vi "SMS Analysis Interface User Get Data Path.vi"() -> (4 "Transfer Log Path":string, 6 "Image Name":string, 8 "Frames":u32, 10 "Cycles":u16, 15 "Error":errorcluster)   [LabVIEW 2016]
uses:
  Tools/Metadata/Microscope Metadata/Device Metadata Types/Capture Metadata.ctl
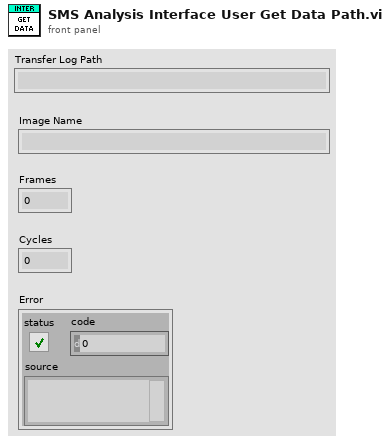
[diagram p1: front panel]
types:
  T1 = typedef "Capture Metadata.ctl" = cluster{"Capture_Exposure_sec":dbl, "Cycles":u16, "Frames":u32, "No_of_Z_Steps":u16, "Z_Step_Size_um":dbl, "Init_Z_Position_um":dbl, "Save_Path":string, "Line_Scan":bool, "Line_Scan_Mode":string}
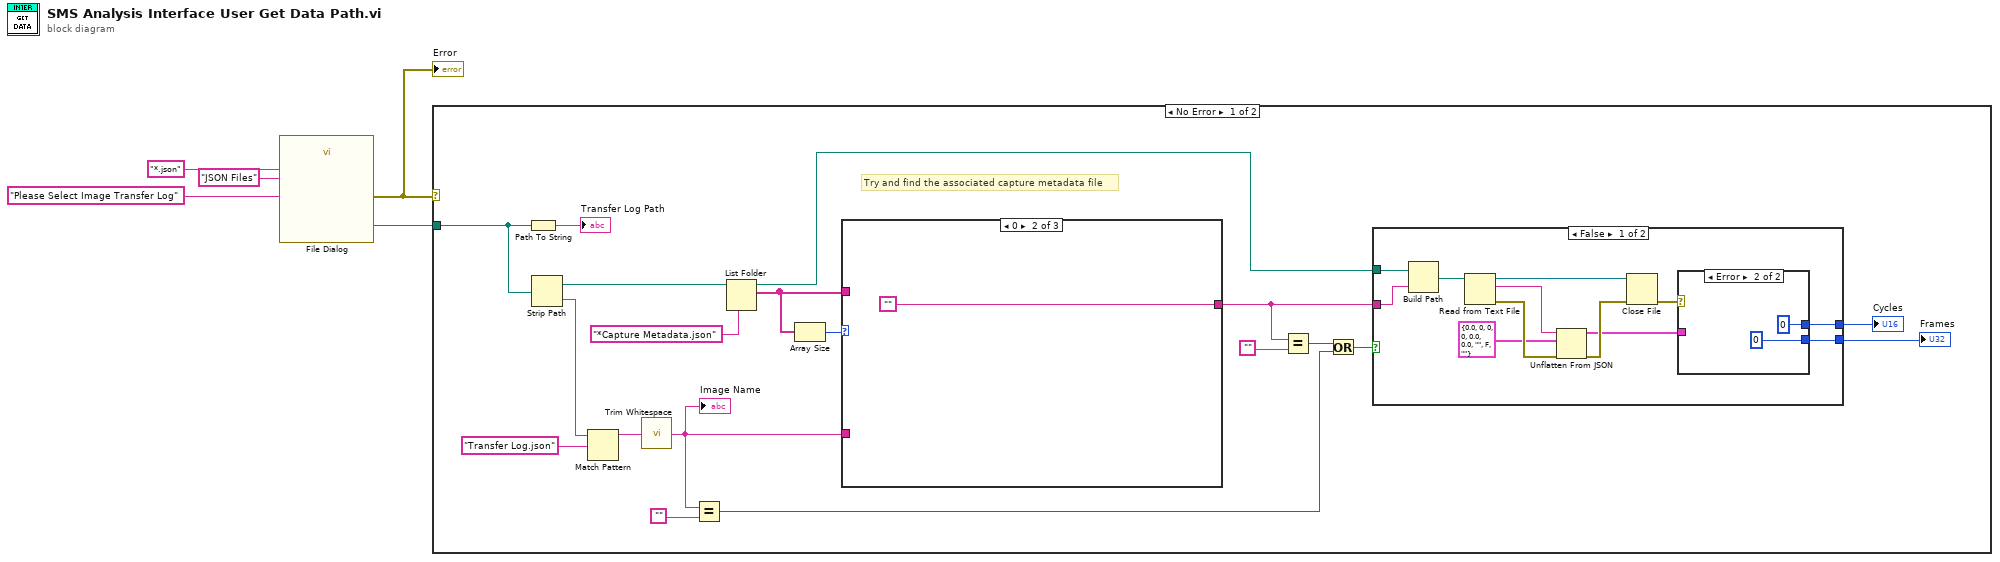
[diagram p0: block diagram]
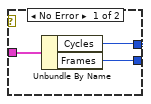
[diagram p2: hidden frame]
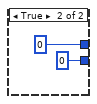
[diagram p3: hidden frame]
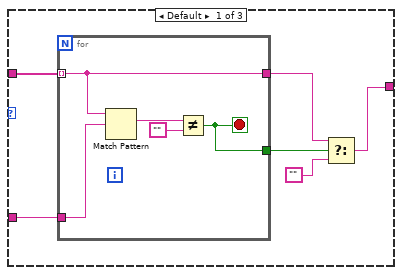
[diagram p4: hidden frame]
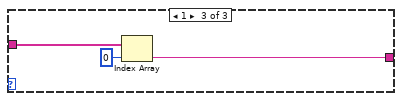
[diagram p5: hidden frame]
diagram:
  n1 = call "File Dialog"("prompt"="Please Select Image Transfer Log", "pattern (all files)"="*.json", "pattern label"="JSON Files") -> ("selected path"=w2:path, "error out"=w1:errorcluster)  [unwired: 9 in, 2 out]
  "Error" <- w1
  n2 = case shown="No Error" w1 {
    tunnel: w2 -> [w23 _]
    frame No Error {
      # "Try and find the associated capture metadata file"
      n3 = Path To String(path=w23) -> (string=→"Transfer Log Path":string)
      n4 = Strip Path(path=w23) -> (stripped path=w22:path, name=w19:string)
      n5 = Match Pattern(string=w19, regular expression="Transfer Log.json") -> (before substring=w18:string)  [unwired: 1 in, 3 out]
      n6 = call <vilib>:"Trim Whitespace.vi"("string"=w18) -> ("trimmed string"=w15:string)  [unwired: 1 in]
      "Image Name" <- w15
      n7 = Equal?(x=w15, y="") -> (x = y?=w11:bool)
      n8 = List Folder(path=w22, pattern="*Capture Metadata.json") -> (path out=w8:path, filenames=w16:string[])  [unwired: 2 in, 2 out]
      n9 = Array Size(array=w16) -> (size(s)=w17:i32)
      n10 = case shown="0" w17 {
        tunnel: w16 -> [w49 _ w58]
        tunnel: [w44 "" w56] -> w9
        tunnel: w15 -> [w48 _ _]
        frame Default {
          n11 = for {
            tunnel: w49 -> [w51] mode=indexing
            tunnel: w48 -> [w54]
            tunnel: [w51] -> w46
            tunnel: [w50] -> w47
            stop <- w50 stop-if-true
            n12 = Match Pattern(string=w51, regular expression=w54) -> (match substring=w52:string)  [unwired: 1 in, 3 out]
            n13 = Not Equal?(x=w52, y="") -> (x != y?=w50:bool)
          }
          n14 = Select(t=w46, s=w47, f="") -> (s? t:f=w44:string)
        }
        frame 0 {
        }
        frame 1 {
          n15 = Index Array(array=w58, index=0) -> (element=w56:string)
        }
      }
      n16 = Equal?(x=w9, y="") -> (x = y?=w12:bool)
      n17 = Or(x=w12, y=w11) -> (x .or. y?=w10:bool)
      n18 = case shown="False" w10 {
        tunnel: w9 -> [w35 _]
        tunnel: w8 -> [w36 _]
        tunnel: [w26 u16 0 ("Cycles")] -> w7
        tunnel: [w25 u32 0 ("Frames")] -> w6
        frame False {
          n19 = Build Path(base path=w36, name or relative path=w35) -> (appended path=w34:path)
          n20 = Read from Text File(file (use dialog)=w34) -> (refnum out=w33:refnum<file>, text=w32:string, error out=w31:errorcluster)  [unwired: 3 in, 1 out]
          n21 = Unflatten From JSON(JSON string=w32, type and defaults=T1 {"Capture_Exposure_sec"=0.0, "Cycles"=0, "Frames"=0, "No_of_Z_Steps"=0, "Z_Step_Size_um"=0.0, "Init_Z_Position_um"=0.0, "Save_Path"="", "Line_Scan"=FALSE, "Line_Scan_Mode"=""} ("Capture Metadata"), error in (no error)=w31) -> (value=w27:T1, error out=w30:errorcluster)  [unwired: 4 in]
          n22 = Close File(refnum=w33, error in=w30) -> (error out=w28:errorcluster)  [unwired: 1 out]
          n23 = case shown="Error" w28 {
            tunnel: w27 -> [w39 _]
            tunnel: [w38 u16 0 ("Cycles")] -> w26
            tunnel: [w37 u32 0 ("Frames")] -> w25
            frame No Error {
              n24 = Unbundle By Name(w39) -> ("Cycles"=w38:u16, "Frames"=w37:u32)
            }
            frame Error {
            }
          }
        }
        frame True {
        }
      }
      "Cycles" <- w7
      "Frames" <- w6
    }
    frame Error {
    }
  }
